vi "Measurement Logic.vi"() -> ()   [LabVIEW 2021, in "Single Tone No Gen_Class D Amplifier.lvlib"]
uses:
  Single Tone No Gen_Class D Amplifier.lvlib
  Measurement Configuration.ctl
  shared/controls/weighting filter.ctl
  shared/controls/lowpass filter.ctl
  shared/controls/highpass filter.ctl
  shared/controls/units - snr.ctl
  shared/controls/units - ratio.ctl
  Measurement Results.ctl
  <vilib>/MeasurementLink/MeasurementLink Measurement Server/Measure Call Context/Measure Call Context.lvclass
  shared/controls/single tone audio measurement settings.ctl
  shared/controls/audio filter settings.ctl
  shared/controls/units settings.ctl
  <vilib>/DAQmx/read.llb/DAQmx Read (Analog 1D Wfm NChan NSamp).vi
  <vilib>/DAQmx/create/channels.llb/DAQmx Create Channel (AI-Voltage-Basic).vi
  <vilib>/DAQmx/configure/timing.llb/DAQmx Timing (Sample Clock).vi
  <vilib>/DAQmx/miscellaneous.llb/DAQmx Fill In Error Info.vi
  <vilib>/Waveform/WDTOps.llb/WDT Get Waveform Subset DBL.vi
  shared/controls/audio controls.lvlib
panel:
  out "names out":string[](array[string])
  out "Spectrum":cluster{"x0":dbl, "dx":dbl, "magnitude":dbl[]}[](graph)
  out "Waveform Graph":waveform(dbl)[](graph)=[{"t0"=timestamp(3785336549.595634 s since 1904-01-01), "dt"=1.9531249997269942e-05, "Y"=array[12800 elements], "attributes"=variant("NI_ChannelName"=variant(string "PXI1Slot4/ai0"), "NI_UnitDescription"=variant(string "Volts"))}]
  out "measure call context out":refnum<class "Measure Call Context.lvclass">
  in  "measure call context in":refnum<class "Measure Call Context.lvclass">
  out "measurement results":T1={"channel names"=[], "frequency (Hz)"=[], "amplitude (Vrms)"=[], "amplitude (dBFS)"=[], "phase (deg)"=[], "SNR"=[], "THD+N"=[], "THD"=[], "dynamic range (dB)"=[], "gain"=[], "SFDR (dBc)"=[], "output power (W)"=[], "wfm - t0"=0.0, "wfm - dt"=1.9531249997269942e-05, "wfm - data"=array[12800 elements], "fft - f0"=0.0, "fft - df"=4.000000000559116, "fft - data"=array[6400 elements]}
  in  "measurement configuration":T2={"acq sampling rate"=51200.0, "min measurement cycles"=20, "min measurement time (s)"=0.1, "min settling cycles"=0, "min settling time (s)"=0.005, "acq channel"="PXI1Slot4/ai0", "band start"=20.0, "band stop"=20000.0, "weighting filter"=enum."Linear", "lowpass filter"=enum."No filter", "highpass filter"=enum."DC", "SNR units"=enum."dB", "THD+N units"=enum."dB", "THD units"=enum."dB", "gain units"=enum."dB", "expected amplitude (Vpk)"=2.0, "signal frequency"=2000.0, "amplitude reference (Vpk-pk)"=15.0, "load impedance"=4.0} {"signal frequency" format="%#_13g"; "min settling time (s)" format="%.0p"; "min measurement time (s)" format="%.0p"; "min measurement cycles" format="%#_6p"; "band stop" format="%#_6pHz"; "band start" format="%#_6pHz"; "acq sampling rate" format="%0.2f"}
  out "error out":errorcluster
  in  "error in":errorcluster
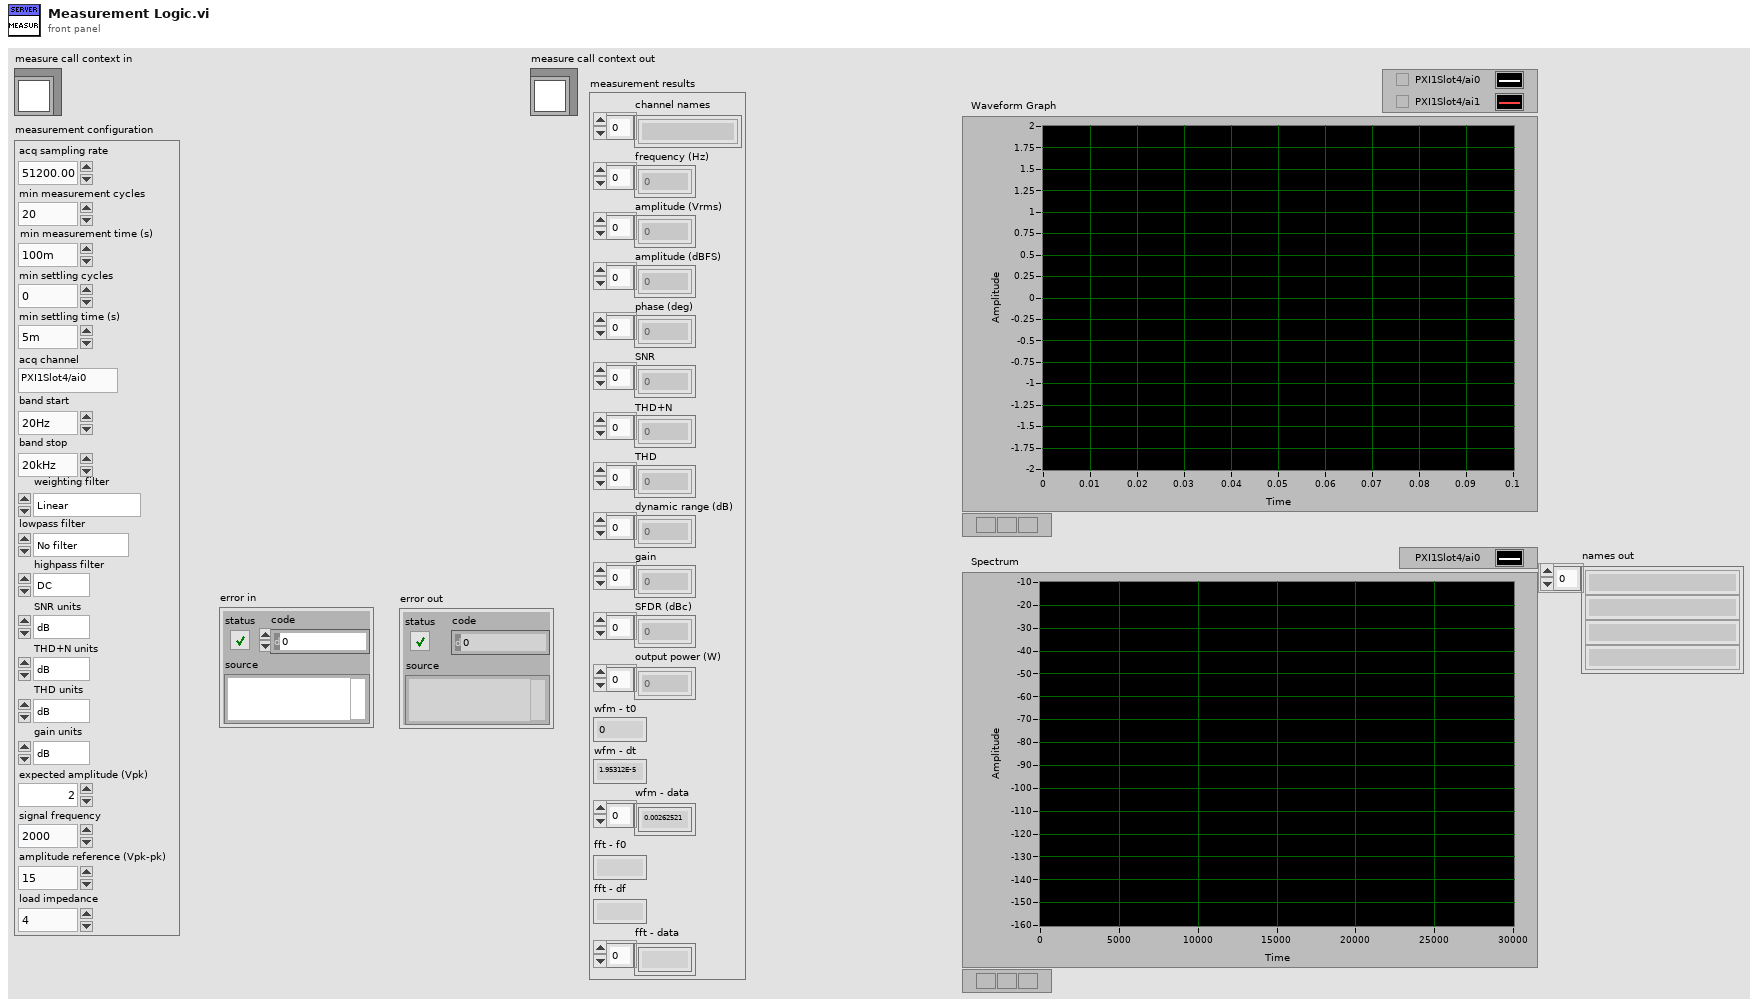
[diagram p1: front panel]
types:
  T1 = typedef "Single Tone No Gen_Class D Amplifier.lvlib/Measurement Results.ctl" = cluster{"channel names":string[], "frequency (Hz)":dbl[], "amplitude (Vrms)":dbl[], "amplitude (dBFS)":dbl[], "phase (deg)":dbl[], "SNR":dbl[], "THD+N":dbl[], "THD":dbl[], "dynamic range (dB)":dbl[], "gain":dbl[], "SFDR (dBc)":dbl[], "output power (W)":dbl[], "wfm - t0":dbl, "wfm - dt":dbl, "wfm - data":dbl[], "fft - f0":dbl, "fft - df":dbl, "fft - data":dbl[]}
  T2 = typedef "Single Tone No Gen_Class D Amplifier.lvlib/Measurement Configuration.ctl" = cluster{"acq sampling rate":dbl, "min measurement cycles":u32, "min measurement time (s)":dbl, "min settling cycles":u32, "min settling time (s)":dbl, "acq channel":string, "band start":dbl, "band stop":dbl, "weighting filter":T3, "lowpass filter":T4, "highpass filter":T5, "SNR units":T6, "THD+N units":T7, "THD units":T7, "gain units":T7, "expected amplitude (Vpk)":dbl, "signal frequency":dbl, "amplitude reference (Vpk-pk)":dbl, "load impedance":dbl}
  T3 = typedef "weighting filter.ctl" = enum32{"Linear", "A-weighting", "B-weighting", "C-weighting"}
  T4 = typedef "lowpass filter.ctl" = enum32{"No filter", "AES17 20kHz", "AES17 40kHz"}
  T5 = typedef "highpass filter.ctl" = enum32{"DC", "AC"}
  T6 = typedef "audio controls.lvlib/units - snr.ctl" = enum32{"dB", "x/y"}
  T7 = typedef "audio controls.lvlib/units - ratio.ctl" = enum32{"dB", "%", "x/y"}
  T8 = typedef "audio controls.lvlib/units settings.ctl" = cluster{"SNR units":T6, "THD+N units":T7, "THD units":T7, "gain units":T7}
  T9 = typedef "audio filter settings.ctl" = cluster{"weighting filter":T3, "highpass filter":T5, "lowpass filter ":T4}
  T10 = typedef "single tone audio measurement settings.ctl" = cluster{"Band start":dbl, "Band stop":dbl, "Amplitude":dbl, "Frequency":dbl, "Full scale range":dbl}
  T11 = typedef "audio controls.lvlib/single tone audio measurements.ctl" = cluster{"channel":string, "frequency (Hz)":dbl, "amplitude (Vrms)":dbl, "amplitude (dBFS)":dbl, "phase (deg)":dbl, "SNR":dbl, "THD+N":dbl, "THD":dbl, "dynamic range (dB)":dbl, "gain":dbl, "SFDR (dBc)":dbl}
  T12 = typedef "audio controls.lvlib/single tone audio measurements (N chan).ctl" = cluster{"channel names":string[], "frequency (Hz)":dbl[], "amplitude (Vrms)":dbl[], "amplitude (dBFS)":dbl[], "phase (deg)":dbl[], "SNR":dbl[], "THD+N":dbl[], "THD":dbl[], "dynamic range (dB)":dbl[], "gain":dbl[], "SFDR (dBc)":dbl[]}
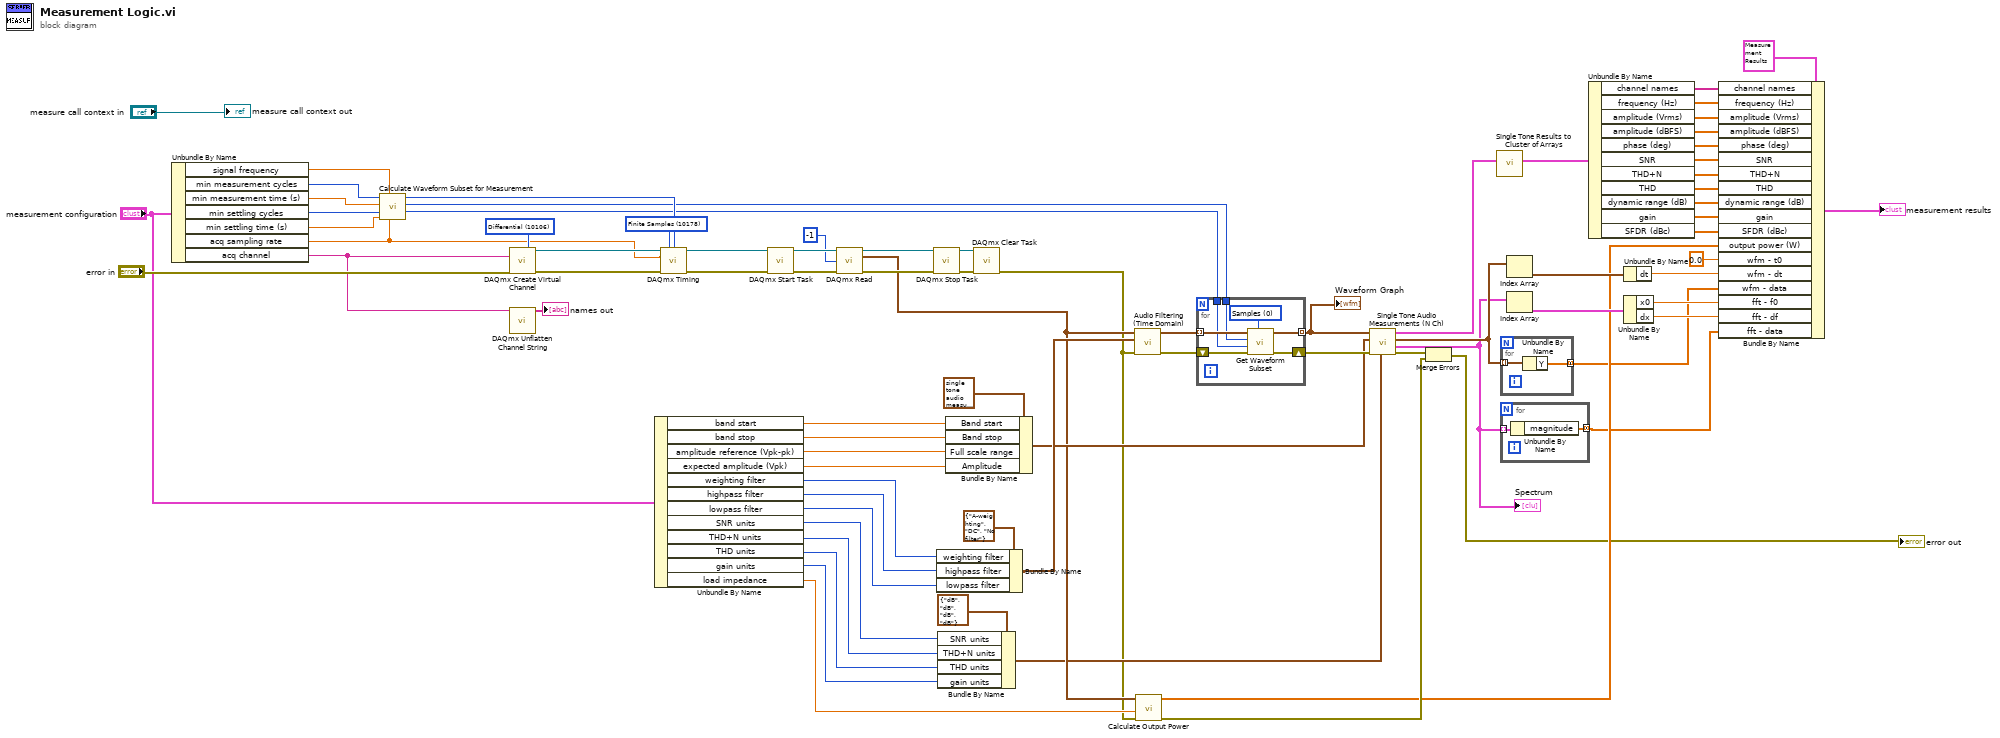
[diagram p0: block diagram]
diagram:
  w64 = 10106 items=["Default"=-1, "RSE"=10083, "NRSE"=10078, "Differential"=10106, "Pseudodifferential"=12529] ("input terminal configuration")
  w69 = 10178 items=["Finite Samples"=10178, "Continuous Samples"=10123, "Hardware Timed Single Point"=12522] ("sample mode")
  n1 = Unbundle By Name("measurement configuration") -> ("signal frequency"=w44:dbl, "min measurement cycles"=w48:u32, "min measurement time (s)"=w47:dbl, "min settling cycles"=w46:u32, "min settling time (s)"=w45:dbl, "acq sampling rate"=w42:dbl, "acq channel"=w27:string)
  n2 = call "Calculate Waveform Subset for Measurement.vi"("sampling rate"=w42, "signal frequency"=w44, "minimum settling duration"=w45, "minimum settling cycles"=w46, "minimum measurement duration"=w47, "minimum measurement cycles"=w48) -> ("duration (samples)"=w39:u32, "start (samples)"=w40:u32, "total acquisition (samples)"=w41:u32)  [unwired: 3 in]
  n3 = call-poly <vilib>:"DAQmx Create Virtual Channel.vi"("input terminal configuration"=w64, "physical channels"=w27, "error in"="error in") -> ("task out"=w78:refnum<k21>, "error out"=w79:errorcluster)  [unwired: 11 in]
  n4 = call <vilib>:"DAQmx Unflatten Channel String.vi"("names in"=w27) -> ("names out"=→"names out":string[])  [unwired: 13 in, 1 out]
  n5 = Unbundle By Name("measurement configuration") -> ("band start"=w56:dbl, "band stop"=w55:dbl, "amplitude reference (Vpk-pk)"=w49:dbl, "expected amplitude (Vpk)"=w1:dbl, "weighting filter"=w2:T3, "highpass filter"=w53:T5, "lowpass filter"=w52:T4, "SNR units"=w35:T6, "THD+N units"=w34:T7, "THD units"=w33:T7, "gain units"=w32:T7, "load impedance"=w36:dbl)
  n6 = call-poly <vilib>:"DAQmx Timing.vi"("task/channels in"=w78, "sample mode"=w69, "samples per channel"=w41, "rate"=w42, "error in"=w79) -> ("task out"=w70:refnum<k21>, "error out"=w4:errorcluster)  [unwired: 9 in]
  n7 = call <vilib>:"DAQmx Start Task.vi"("task/channels in"=w70, "error in"=w4) -> ("task out"=w73:refnum<k21>, "error out"=w76:errorcluster)  [unwired: 12 in]
  n8 = call-poly <vilib>:"DAQmx Read.vi"("task/channels in"=w73, "number of samples per channel"=-1, "error in"=w76) -> ("task out"=w72:refnum<k21>, "data"=w43:waveform(dbl)[], "error out"=w75:errorcluster)  [unwired: 10 in]
  n9 = call <vilib>:"DAQmx Stop Task.vi"("task/channels in"=w72, "error in"=w75) -> ("task out"=w77:refnum<k21>, "error out"=w74:errorcluster)  [unwired: 12 in]
  n10 = Bundle By Name(cluster=T9 {"weighting filter"=enum."A-weighting", "highpass filter"=enum."DC", "lowpass filter "=enum."No filter"} ("filter settings"), "weighting filter"=w2, "highpass filter"=w53, "lowpass filter"=w52) -> (w51:T9)
  n11 = Bundle By Name(cluster=T8 {"SNR units"=enum."dB", "THD+N units"=enum."dB", "THD units"=enum."dB", "gain units"=enum."dB"} ("units settings"), "SNR units"=w35, "THD+N units"=w34, "THD units"=w33, "gain units"=w32) -> (w37:T8)
  n12 = Bundle By Name(cluster=T10 {"Band start"=20.0, "Band stop"=20000.0, "Amplitude"=-1.0, "Frequency"=1000.0, "Full scale range"=15.0} ("measurement settings"), "Band start"=w56, "Band stop"=w55, "Full scale range"=w49, "Amplitude"=w1) -> (w50:T10)
  n13 = call <vilib>:"DAQmx Clear Task.vi"("task in"=w77, "error in"=w74) -> ("error out"=w31:errorcluster)  [unwired: 13 in]
  n14 = call "Audio Filtering (Time Domain).vi"("waveforms"=w43, "filter settings"=w51, "error in"=w31) -> ("time domain"=w60:waveform(dbl)[], "error out"=w61:errorcluster)  [unwired: 6 in]
  n15 = call "Calculate Output Power.vi"("error in (no error)"=w31, "load impedance"=w36, "waveforms"=w43) -> ("error out"=w62:errorcluster, "output power"=w10:dbl[])  [unwired: 7 in]
  n16 = for {
    tunnel: w60 -> [w87] mode=indexing
    tunnel: [w86] -> w30 mode=indexing
    shift-right: [w83] -> w59
    shift-left: w61 -> [w84]
    tunnel: w40 -> [w82]
    tunnel: w39 -> [w81]
    w85 = u16 0 items=["Samples", "Relative Time"] ("start/duration format")
    n17 = call-poly <vilib>:"Get Waveform Subset.vi"("start/duration format"=w85, "error in (no error)"=w84, "duration"=w81, "start samples/time"=w82, "waveform in"=w87) -> ("error out"=w83:errorcluster, "waveform out"=w86:waveform(dbl))  [unwired: 1 in, 2 out]
  }
  "Waveform Graph" <- w30
  n18 = call "Single Tone Audio Measurements (N Ch).vi"("units settings"=w37, "error in"=w59, "measurement settings"=w50, "waveforms"=w30) -> ("error out"=w58:errorcluster, "spectra"=w8:cluster{"x0":dbl, "dx":dbl, "magnitude":dbl[]}[], "waveforms"=w9:waveform(dbl)[], "results"=w23:T11[])  [unwired: 4 in]
  "Spectrum" <- w8
  n19 = Merge Errors(w58, w62) -> (→"error out":errorcluster)
  n20 = call "Single Tone Results to Cluster of Arrays.vi"("results"=w23) -> ("results (N chan)"=w22:T12)  [unwired: 10 in]
  n21 = for {
    tunnel: w8 -> [w89] mode=indexing
    tunnel: [w88] -> w7 mode=concatenating
    n22 = Unbundle By Name(w89) -> ("magnitude"=w88:dbl[])
  }
  n23 = for {
    tunnel: w9 -> [w91] mode=indexing
    tunnel: [w90] -> w6 mode=concatenating
    n24 = Unbundle By Name(w91) -> ("Y"=w90:dbl[])
  }
  n25 = Index Array(array=w9) -> (element=w29:waveform(dbl))  [unwired: 1 in]
  n26 = Index Array(array=w8) -> (element=w28:cluster{"x0":dbl, "dx":dbl, "magnitude":dbl[]})  [unwired: 1 in]
  n27 = Unbundle By Name(w22) -> ("channel names"=w21:string[], "frequency (Hz)"=w20:dbl[], "amplitude (Vrms)"=w19:dbl[], "amplitude (dBFS)"=w18:dbl[], "phase (deg)"=w17:dbl[], "SNR"=w16:dbl[], "THD+N"=w15:dbl[], "THD"=w14:dbl[], "dynamic range (dB)"=w13:dbl[], "gain"=w12:dbl[], "SFDR (dBc)"=w11:dbl[])
  n28 = Unbundle By Name(w29) -> ("dt"=w67:dbl)
  n29 = Unbundle By Name(w28) -> ("x0"=w66:dbl, "dx"=w65:dbl)
  n30 = Bundle By Name(cluster=T1 {"channel names"=[], "frequency (Hz)"=[], "amplitude (Vrms)"=[], "amplitude (dBFS)"=[], "phase (deg)"=[], "SNR"=[], "THD+N"=[], "THD"=[], "dynamic range (dB)"=[], "gain"=[], "SFDR (dBc)"=[], "output power (W)"=[], "wfm - t0"=0.0, "wfm - dt"=0.0, "wfm - data"=[], "fft - f0"=0.0, "fft - df"=0.0, "fft - data"=[]} ("Measurement Results"), "channel names"=w21, "frequency (Hz)"=w20, "amplitude (Vrms)"=w19, "amplitude (dBFS)"=w18, "phase (deg)"=w17, "SNR"=w16, "THD+N"=w15, "THD"=w14, "dynamic range (dB)"=w13, "gain"=w12, "SFDR (dBc)"=w11, "output power (W)"=w10, "wfm - t0"=0.0, "wfm - dt"=w67, "wfm - data"=w6, "fft - f0"=w66, "fft - df"=w65, "fft - data"=w7) -> (→"measurement results":T1)
  "measure call context out" <- "measure call context in"
